vi "Two Camera Track and Save v1.vi"() -> ()   [LabVIEW 2014]
uses:
  <vilib>/vision/Image Controls.llb/IMAQ Image.ctl
  <vilib>/Platform/TimedLoop/XDataNode/timing_clust.ctl
  <vilib>/Platform/TimedLoop/XDataNode/nitl_modes.ctl
  <vilib>/Platform/TimedLoop/XDataNode/wakeup.ctl
  <vilib>/event_ctls.llb/eventvkey.ctl
  <vilib>/userdefined/High Color/IMAQdx.ctl
  <vilib>/platform/TimedLoop/XDataNode/XDataNode.xnode
  <vilib>/vision/driver/NI_Vision_Acquisition_Software.lvlib
  <vilib>/Platform/TimedLoop/XDataNode/XDNodeRunTimeDep.lvlib
panel:
  in  "Comments 2":string
  out "Cam2 Dropped Frames":u32
  out "Cam2 Dropped Hidden":u32 caption="Dropped Frames"
  out "Written":string
  in  "Comments":string
  out "User Comments  File":path
  out "Centroid File Path":path
  out "Cam2 AVI File Path":path
  out "Cam1 AVI File Path":path
  out "Save Directory":path
  out "Time Elapsed (H : M : S)":string
  out "Cam1 Dropped Frames":u32
  out "Cam1 Composite Out":T1
  out "Cam2 Composite Out":T1
  out "Cam2 Composite":T1(plugin-control)
  out "Cam1 Composite":T1(plugin-control)
  in  "Save to AVI":bool
  out "Cam1 Dropped Hidden":u32 caption="Dropped Frames"
  in  "Image Threshold Range":cluster{"Lower Value":dbl, "Upper Value":dbl}={"Lower Value"=0.0, "Upper Value"=80.0}
  in  "stop":bool
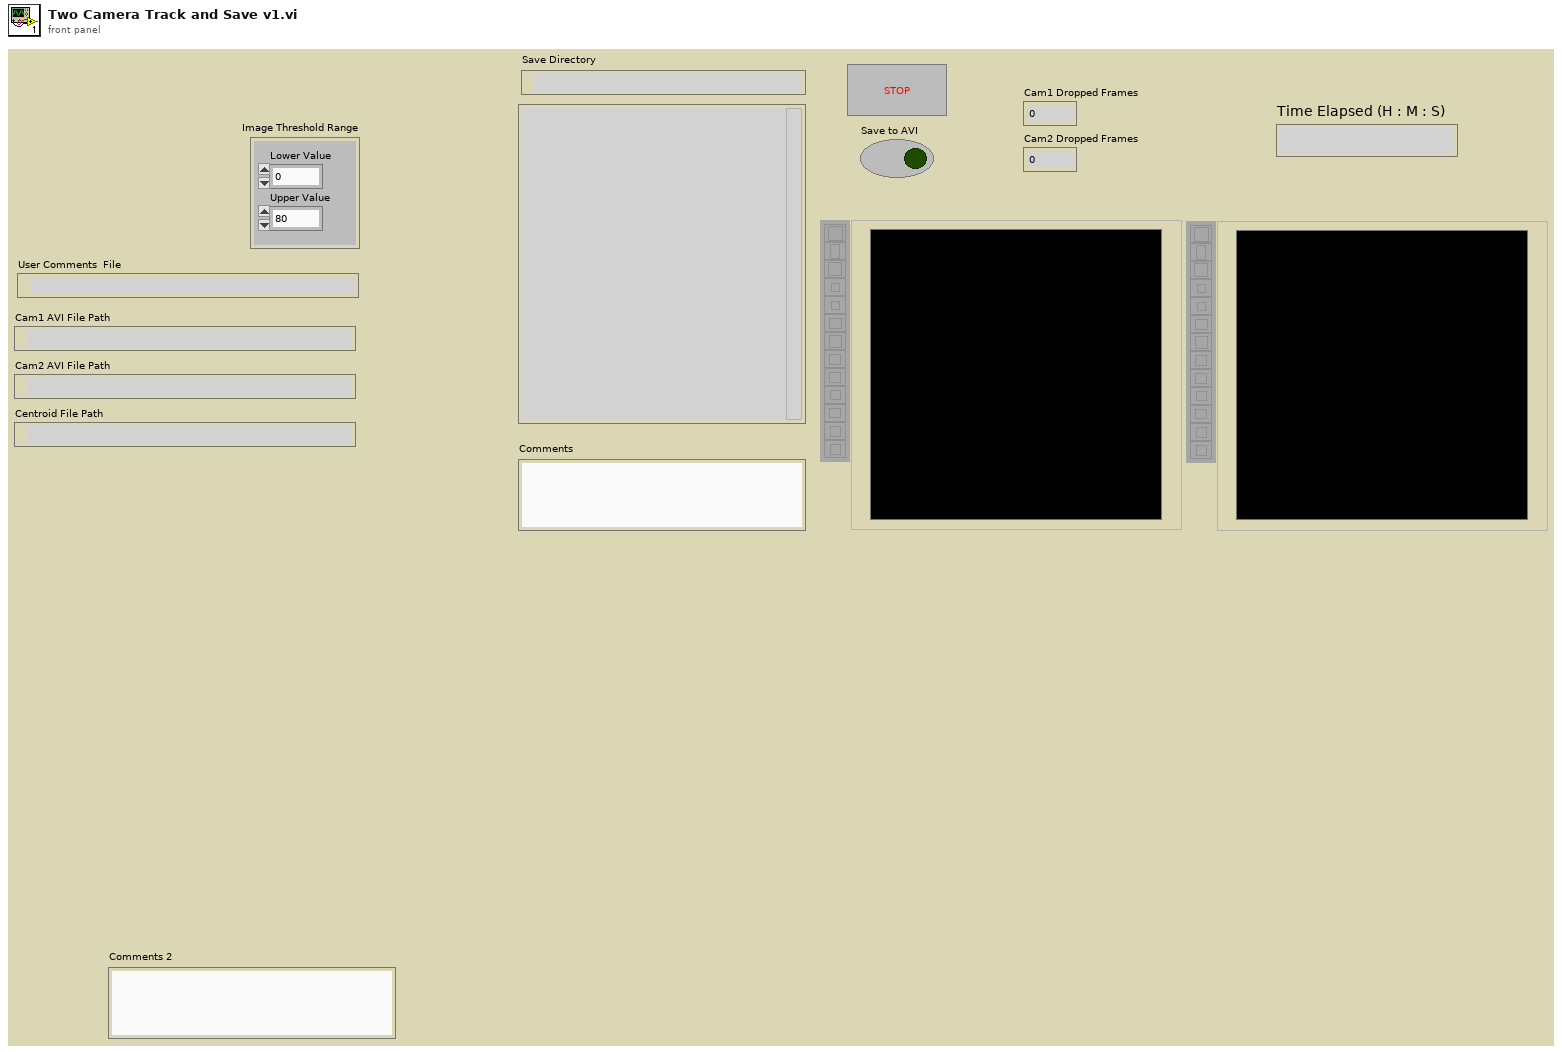
[diagram p1: front panel]
types:
  T1 = typedef "IMAQ Image.ctl" = refnum<image>
  T2 = enum16{"open", "replace", "create", "open or create", "replace or create", "replace or create with confirmation"}
  T3 = typedef "IMAQdx.ctl" = refnum<k21>
  T4 = typedef "AviRefnum.ctl" = refnum<k1>
  T5 = typedef "XDNodeRunTimeDep.lvlib/timing_clust.ctl" = cluster{"Expected End [f-1]":u64, "Actual End [f-1]":u64, "Finished Late? [f-1]":bool, "Expected End [i-1]":u64, "Actual End [i-1]":u64, "Finished Late? [i-1]":bool, "Expected Start [i]":u64, "Actual Start [i]":u64, "Expected Start [f]":u64, "Actual Start [f]":u64, "Source Name":string, "Structure Name":string, "Period":i64, "Deadline":i64, "Offset":i64, "Start":i64, "Priority":i32, "Timeout":i32, "Mode":T6, "Wakeup Reason":T7, "Error":errorcluster, "Source Type":string, "Secondary Source Type":string, "Global End Time":u64, "Global Start Time":u64, "Frame Duration":u64, "Iteration Duration":u64, "Assigned CPU":i32, "I/O Scan Engine Mode":u32}
  T6 = typedef "XDNodeRunTimeDep.lvlib/nitl_modes.ctl" = enum32{"No Change", "Process missed periods, maintain original phase", "Discard missed periods, maintain original phase", "Process missed periods, ignore original phase", "Discard missed periods, ignore original phase"}
  T7 = typedef "XDNodeRunTimeDep.lvlib/wakeup.ctl" = enum32{"Normal", "Aborted", "Asynchronous wakeup", "Timing source error", "Timed loop error", "Timeout"}
  T8 = typedef "eventvkey.ctl" = enum16{"ASCII", "Enter", "Return", "Shift", "Ctrl", "Alt", "Cmd", "Opt", "Caps", "NumLock", "Clear", "Break", "Up", "Down", "Left", "Right", "Insert", "Delete", "Home", "End", "PageUp", "PageDown", "Escape", "Help", "Pause", "ScrollLock", "F1", "F2", "F3", "F4", "F5", "F6", "F7", "F8", "F9", "F10", "F11", "F12", "F13", "F14", "F15", "F16", "F17", "F18", "F19", "F20", "F21", "F22", "F23", "F24", "Play", "VolumeUp", "VolumeDown", "Mute", "Two Byte Char"}
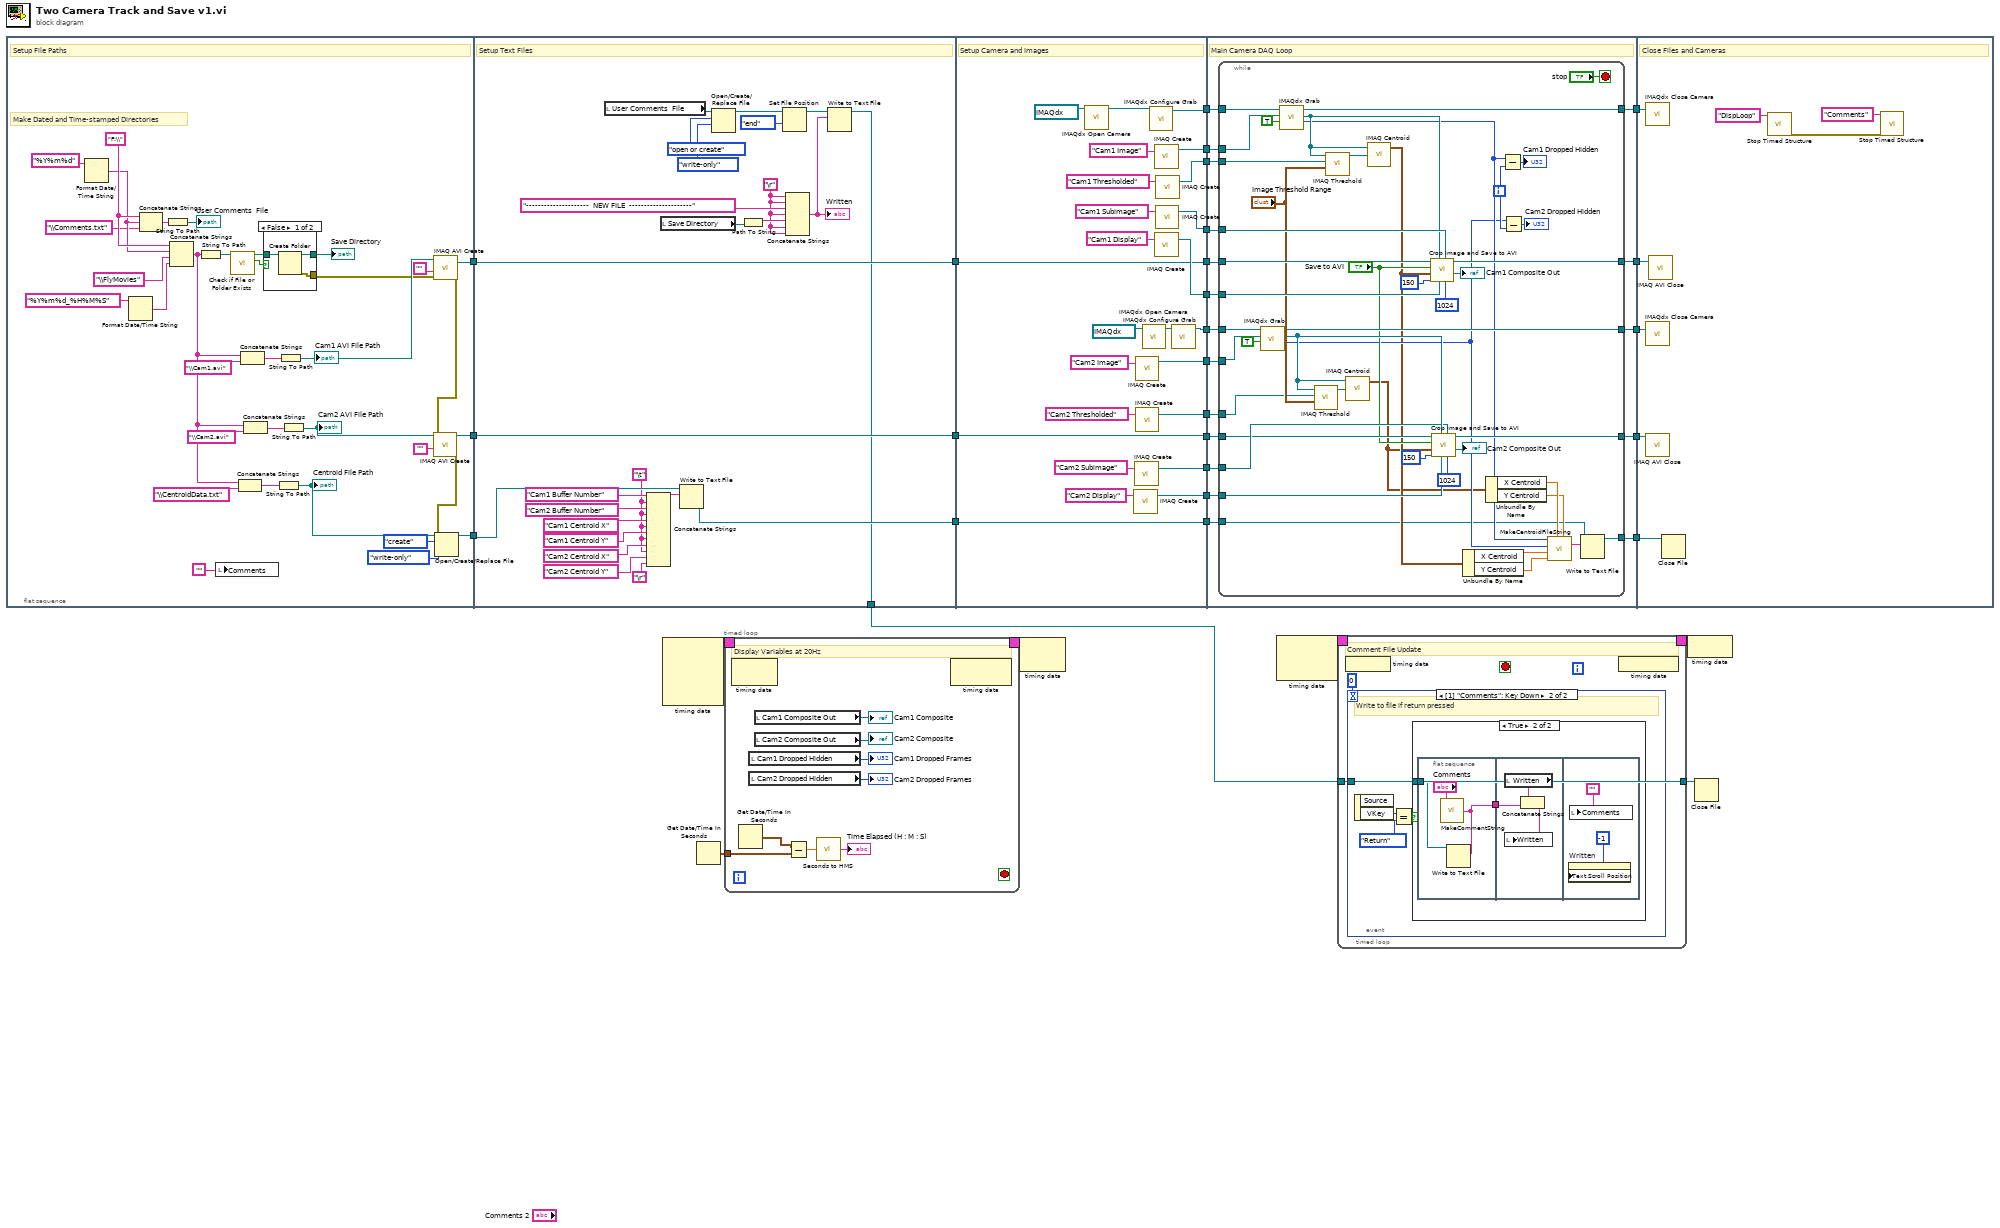
[diagram p0: block diagram]
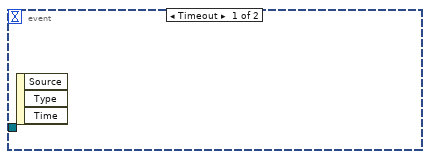
[diagram p2: hidden frame]
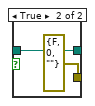
[diagram p4: hidden frame]
diagram:
  n1 = flat-sequence {
    tunnel: [w65] -> w12
    tunnel: [w64] -> w10
    tunnel: [w39] -> w8
    tunnel: w12 -> [w95]
    tunnel: [w95] -> w11
    tunnel: w10 -> [w94]
    tunnel: [w94] -> w9
    tunnel: w8 -> [w79]
    tunnel: [w77] -> w7
    tunnel: [w71] -> w1
    tunnel: [w116] -> w24
    tunnel: [w117] -> w23
    tunnel: [w112] -> w22
    tunnel: [w111] -> w21
    tunnel: [w109] -> w20
    tunnel: [w106] -> w19
    tunnel: [w105] -> w18
    tunnel: [w101] -> w17
    tunnel: [w100] -> w16
    tunnel: [w99] -> w15
    tunnel: [w97] -> w14
    tunnel: w11 -> [w98]
    tunnel: [w98] -> w13
    tunnel: w9 -> [w97]
    tunnel: w7 -> [w96]
    tunnel: [w96] -> w6
    tunnel: [w136] -> w31
    tunnel: w24 -> [w138]
    tunnel: w23 -> [w137]
    tunnel: w22 -> [w135]
    tunnel: w21 -> [w134]
    tunnel: [w133] -> w30
    tunnel: w20 -> [w132]
    tunnel: [w130] -> w29
    tunnel: w19 -> [w129]
    tunnel: w18 -> [w128]
    tunnel: w14 -> [w127]
    tunnel: w17 -> [w126]
    tunnel: w16 -> [w125]
    tunnel: w15 -> [w124]
    tunnel: [w123] -> w28
    tunnel: w13 -> [w131]
    tunnel: w6 -> [w122]
    tunnel: [w121] -> w5
    tunnel: w31 -> [w191]
    tunnel: w30 -> [w190]
    tunnel: w29 -> [w189]
    tunnel: w28 -> [w188]
    tunnel: w5 -> [w186]
    frame #0 {
      w46 = "F:\\"
      # "Make Dated and Time-stamped Directories"
      # "Setup File Paths"
      n2 = Format Date/Time String(time format string (%c)="%Y%m%d") -> (date/time string=w45:string)  [unwired: 2 in]
      n3 = Format Date/Time String(time format string (%c)="%Y%m%d_%H%M%S") -> (date/time string=w58:string)  [unwired: 2 in]
      n4 = Concatenate Strings(w46, w45, "\\Comments.txt" ("string")) -> (w43:string)
      n5 = String To Path(string=w43) -> (path=→"User Comments  File":path)
      n6 = Concatenate Strings(w46, w45, "\\FlyMovies", w58) -> (w48:string)
      n7 = String To Path(string=w48) -> (path=w57:path)
      n8 = local write "Comments"("") -> ()
      n9 = call <vilib>:"Check if File or Folder Exists.vi"("path"=w57) -> ("file or folder exists?"=w62:bool, "dup path"=w61:path)  [unwired: 8 in, 1 out]
      n10 = Concatenate Strings(w48, "\\CentroidData.txt" ("string")) -> (w51:string)
      n11 = Concatenate Strings(w48, "\\Cam1.avi" ("string")) -> (w54:string)
      n12 = Concatenate Strings(w48, "\\Cam2.avi" ("string")) -> (w53:string)
      n13 = case shown="False" w62 {
        tunnel: [w67 w70] -> w56
        tunnel: w61 -> [w68 w70]
        tunnel: [w66 errorcluster {"status"=FALSE, "code"=0, "source"=""} ("error out")] -> w36
        frame False {
          n14 = Create Folder(path (use dialog)=w68) -> (created path=w67:path, error out=w66:errorcluster)  [unwired: 2 in, 1 out]
        }
        frame True {
        }
      }
      "Save Directory" <- w56
      n15 = String To Path(string=w51) -> (path=w40:path)
      "Centroid File Path" <- w40
      n16 = String To Path(string=w54) -> (path=w42:path)
      "Cam1 AVI File Path" <- w42
      n17 = String To Path(string=w53) -> (path=w41:path)
      "Cam2 AVI File Path" <- w41
      n18 = call "IMAQ AVI Create"("error in (no error)"=w36, "Compression Filter"="", "AVI Path"=w42) -> ("error out"=w35:errorcluster, "Avi Refnum"=w65:T4)  [unwired: 7 in]
      n19 = call "IMAQ AVI Create"("error in (no error)"=w35, "Compression Filter"="", "AVI Path"=w41) -> ("error out"=w34:errorcluster, "Avi Refnum"=w64:T4)  [unwired: 7 in]
      n20 = Open/Create/Replace File(file path (use dialog)=w40, error in=w34, operation (0:open)=T2."create", access (0:read/write)=enum16{"read/write", "read-only", "write-only"}."write-only") -> (refnum out=w39:refnum<file>)  [unwired: 2 in, 2 out]
    }
    frame #1 {
      w74 = "\t"
      w86 = "\r"
      # "Setup Text Files"
      n21 = local read "User Comments  File"() -> (w84:path)
      n22 = Concatenate Strings("Cam1 Buffer Number", w74, "Cam2 Buffer Number", w74, "Cam1 Centroid X", w74, "Cam1 Centroid Y", w74, "Cam2 Centroid X", w74, "Cam2 Centroid Y", "\r") -> (w78:string)
      n23 = local read "Save Directory"() -> (w83:path)
      n24 = Write to Text File(file (use dialog)=w79, text=w78) -> (refnum out=w77:refnum<file>)  [unwired: 2 in, 2 out]
      n25 = Open/Create/Replace File(file path (use dialog)=w84, operation (0:open)=T2."open or create", access (0:read/write)=enum16{"read/write", "read-only", "write-only"}."write-only") -> (refnum out=w91:refnum<file>)  [unwired: 3 in, 2 out]
      n26 = Path To String(path=w83) -> (string=w87:string)
      n27 = Set File Position(refnum=w91, from (0:start)=enum16{"start", "end", "current"}."end") -> (refnum out=w89:refnum<file>)  [unwired: 2 in, 1 out]
      n28 = Concatenate Strings(w86, w86, "---------------------  NEW FILE  ---------------------", w86, w87, w86, w86) -> (w85:string)
      "Written" <- w85
      n29 = Write to Text File(file (use dialog)=w89, text=w85) -> (refnum out=w71:refnum<file>)  [unwired: 2 in, 2 out]
    }
    frame #2 {
      # "Setup Camera and Images"
      n30 = call <vilib>:"IMAQdx Open Camera.vi"("Session In"=T3 "cam1") -> ("Session Out"=w119:T3)  [unwired: 9 in, 1 out]
      n31 = call "IMAQ Create"("Image Name"="Cam2 Display") -> ("New Image"=w99:T1)  [unwired: 4 in, 1 out]
      n32 = call "IMAQ Create"("Image Name"="Cam2 Subimage") -> ("New Image"=w100:T1)  [unwired: 4 in, 1 out]
      n33 = call "IMAQ Create"("Image Name"="Cam2 Image") -> ("New Image"=w112:T1)  [unwired: 4 in, 1 out]
      n34 = call "IMAQ Create"("Image Name"="Cam2 Thresholded") -> ("New Image"=w101:T1)  [unwired: 4 in, 1 out]
      n35 = call <vilib>:"IMAQdx Open Camera.vi"("Session In"=T3 "cam3") -> ("Session Out"=w114:T3)  [unwired: 9 in, 1 out]
      n36 = call <vilib>:"IMAQdx Configure Grab.vi"("Session In"=w119) -> ("Session Out"=w116:T3)  [unwired: 9 in, 1 out]
      n37 = call "IMAQ Create"("Image Name"="Cam1 Image") -> ("New Image"=w117:T1)  [unwired: 4 in, 1 out]
      n38 = call "IMAQ Create"("Image Name"="Cam1 Display") -> ("New Image"=w105:T1)  [unwired: 4 in, 1 out]
      n39 = call "IMAQ Create"("Image Name"="Cam1 Subimage") -> ("New Image"=w106:T1)  [unwired: 4 in, 1 out]
      n40 = call "IMAQ Create"("Image Name"="Cam1 Thresholded") -> ("New Image"=w109:T1)  [unwired: 4 in, 1 out]
      n41 = call <vilib>:"IMAQdx Configure Grab.vi"("Session In"=w114) -> ("Session Out"=w111:T3)  [unwired: 9 in, 1 out]
    }
    frame #3 {
      # "Main Camera DAQ Loop"
      n42 = while {
        tunnel: w138 -> [w183]
        tunnel: w137 -> [w182]
        tunnel: [w180] -> w136
        tunnel: w135 -> [w177]
        tunnel: w134 -> [w178]
        tunnel: [w165] -> w133
        tunnel: w132 -> [w174]
        tunnel: w131 -> [w172]
        tunnel: [w171] -> w130
        tunnel: w129 -> [w169]
        tunnel: w128 -> [w168]
        tunnel: w127 -> [w156]
        tunnel: w126 -> [w164]
        tunnel: w125 -> [w158]
        tunnel: w124 -> [w157]
        tunnel: [w154] -> w123
        tunnel: w122 -> [w140]
        tunnel: [w139] -> w121
        i -> [w150]
        stop <- "stop" stop-if-true
        n43 = call <vilib>:"IMAQdx Grab.vi"("Wait for Next Buffer? (Yes)"=TRUE, "Image In"=w177, "Session In"=w178) -> ("Buffer Number Out"=w148:u32, "Image Out"=w159:T1, "Session Out"=w165:T3)  [unwired: 5 in, 1 out]
        n44 = call <vilib>:"IMAQdx Grab.vi"("Wait for Next Buffer? (Yes)"=TRUE, "Image In"=w182, "Session In"=w183) -> ("Buffer Number Out"=w149:u32, "Image Out"=w162:T1, "Session Out"=w180:T3)  [unwired: 5 in, 1 out]
        n45 = call "IMAQ Threshold"("Range"="Image Threshold Range", "Image Dst"=w164, "Image Src"=w159) -> ("Image Dst Out"=w163:T1)  [unwired: 7 in, 1 out]
        n46 = call "IMAQ Threshold"("Range"="Image Threshold Range", "Image Dst"=w174, "Image Src"=w162) -> ("Image Dst Out"=w175:T1)  [unwired: 7 in, 1 out]
        n47 = call "IMAQ Centroid"("Image Mask"=w163, "Image"=w159) -> ("Centroid"=w144:cluster{"X Centroid":sgl, "Y Centroid":sgl})  [unwired: 2 in, 1 out]
        n48 = call "IMAQ Centroid"("Image Mask"=w175, "Image"=w162) -> ("Centroid"=w147:cluster{"X Centroid":sgl, "Y Centroid":sgl})  [unwired: 2 in, 1 out]
        n49 = call "Crop Image and Save to AVI.vi"("Max Dimension Size (px)"=1024, "ImageDst"=w169, "Image Display"=w168, "Image In"=w162, "Cropped Image Width (px)"=150, "Centroid"=w147, "Record"="Save to AVI", "Avi Refnum In"=w172) -> ("Image Out"=→"Cam1 Composite Out":T1, "Avi Refnum Out"=w171:T4)  [unwired: 2 in]
        n50 = call "Crop Image and Save to AVI.vi"("Max Dimension Size (px)"=1024, "ImageDst"=w158, "Image Display"=w157, "Image In"=w159, "Cropped Image Width (px)"=150, "Centroid"=w144, "Record"="Save to AVI", "Avi Refnum In"=w156) -> ("Image Out"=→"Cam2 Composite Out":T1, "Avi Refnum Out"=w154:T4)  [unwired: 2 in]
        n51 = Unbundle By Name(w147) -> ("X Centroid"=w146:sgl, "Y Centroid"=w145:sgl)
        n52 = Unbundle By Name(w144) -> ("X Centroid"=w143:sgl, "Y Centroid"=w142:sgl)
        n53 = Subtract(x=w149, y=w150) -> (x-y=→"Cam1 Dropped Hidden":u32)
        n54 = Subtract(x=w148, y=w150) -> (x-y=→"Cam2 Dropped Hidden":u32)
        n55 = call "MakeCentroidFileString.vi"("Cam2 Centroid Y"=w142, "Cam2 Centroid X"=w143, "Cam1 Centroid Y"=w145, "Cam1 Centroid X"=w146, "Cam2 Buffer Number"=w148, "Cam1 Buffer Number"=w149) -> ("Output String"=w141:string)  [unwired: 3 in]
        n56 = Write to Text File(file (use dialog)=w140, text=w141) -> (refnum out=w139:refnum<file>)  [unwired: 2 in, 2 out]
      }
    }
    frame #4 {
      # "Close Files and Cameras"
      n57 = call <vilib>:"IMAQdx Close Camera.vi"("Session In"=w191) -> ()  [unwired: 10 in, 1 out]
      n58 = call <vilib>:"IMAQdx Close Camera.vi"("Session In"=w190) -> ()  [unwired: 10 in, 1 out]
      n59 = call "IMAQ AVI Close"("Avi Refnum"=w188) -> ()  [unwired: 10 in, 1 out]
      n60 = call "IMAQ AVI Close"("Avi Refnum"=w189) -> ()  [unwired: 10 in, 1 out]
      n61 = Close File(refnum=w186) -> ()  [unwired: 1 in, 2 out]
      n62 = call <vilib>:"Stop Timed Structure.vi"("name"="DispLoop") -> ("error out"=w184:errorcluster)  [unwired: 10 in]
      n63 = call <vilib>:"Stop Timed Structure.vi"("error in (no error)"=w184, "name"="Comments") -> ()  [unwired: 9 in, 1 out]
    }
  }
  n64 = node-c288() -> (w27:T5)  [unwired: 4 in]
  n65 = Get Date/Time In Seconds() -> (seconds since 1Jan1904=w25:timestamp)
  n66 = timed-loop {
    timing: w27 -> [_]
    timing-out: [_] -> w26
    tunnel: w25 -> [w193]
    stop <- _ stop-if-true
    # "Display Variables at 20Hz"
    n67 = node-c288() -> ()  [unwired: 1 in, 1 out]
    n68 = Get Date/Time In Seconds() -> (seconds since 1Jan1904=w194:timestamp)
    n69 = local read "Cam1 Dropped Hidden"() -> (→"Cam1 Dropped Frames":u32)
    n70 = local read "Cam2 Dropped Hidden"() -> (→"Cam2 Dropped Frames":u32)
    n71 = local read "Cam1 Composite Out"() -> (→"Cam1 Composite":T1)
    n72 = local read "Cam2 Composite Out"() -> (→"Cam2 Composite":T1)
    n73 = Subtract(x=w194, y=w193) -> (x-y=w196:dbl)
    n74 = call "Seconds to HMS.vi"("Time Elapsed in Seconds"=w196) -> ("Time Elapsed (H : M : S)"=→"Time Elapsed (H : M : S)":string)
    n75 = node-c288() -> ()  [unwired: 1 in, 1 out]
  }
  n76 = node-c288(w26) -> ()  [unwired: 1 out]
  n77 = node-c288() -> (w4:T5)  [unwired: 2 in]
  n78 = timed-loop {
    timing: w4 -> [_]
    timing-out: [_] -> w3
    tunnel: w1 -> [w202]
    tunnel: [w202] -> w2
    stop <- _ stop-if-true
    # "Comment File Update"
    n79 = node-c288() -> ()  [unwired: 1 in]
    n80 = event shown="[1] \"Comments\": Key Down" {
      selector: _ -> [_ _]
      dyn-events: _ -> [_ _]
      timeout: 0 -> [_ _]
      tunnel: w202 -> [_ w204]
      event Timeout {
        n81 = event-data() -> ()  [unwired: 1 in, 3 out]
      }
      event "Comments": Key Down {
        # "Write to file if return pressed"
        n82 = event-data() -> ("VKey"=w207:T8)  [unwired: 1 in, 1 out]
        n83 = Equal?(x=w207, y=eventvkey."Return") -> (x = y?=w205:bool)
        n84 = case shown="True" w205 {
          tunnel: w204 -> [_ w208]
          frame False {
          }
          frame True {
            n85 = flat-sequence {
              tunnel: [w212] -> w209
              tunnel: w208 -> [w210]
              tunnel: w209 -> [w215]
              frame #0 {
                n86 = call "MakeCommentString.vi"("Input string"="Comments") -> ("Output String"=w212:string)
                n87 = Write to Text File(file (use dialog)=w210, text=w212) -> ()  [unwired: 2 in, 3 out]
              }
              frame #1 {
                n88 = local read "Written"() -> (w214:string)
                n89 = Concatenate Strings(w214, w215) -> (w213:string)
                n90 = local write "Written"(w213) -> ()
              }
              frame #2 {
                n91 = property on="Written" class="Str"("Text.Scroll Position"=-1) -> ()  [unwired: 2 in, 2 out]
                n92 = local write "Comments"("") -> ()
              }
            }
          }
        }
      }
    }
    n93 = node-c288() -> ()  [unwired: 1 out]
  }
  n94 = node-c288(w3) -> ()
  n95 = Close File(refnum=w2) -> ()  [unwired: 1 in, 2 out]
